vi "calculate Y ref.vi"(10 "Step size Y":dbl, 11 "Scan Index":i32) -> (2 "Next_Y_ref":dbl, 3 "Y_ref":dbl)   [LabVIEW 2014]
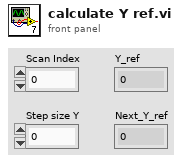
[diagram p1: front panel]
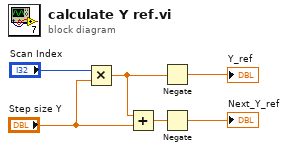
[diagram p0: block diagram]
diagram:
  n1 = Multiply(x="Scan Index", y="Step size Y") -> (x*y=w4:dbl)
  n2 = Add(x=w4, y="Step size Y") -> (x+y=w2:dbl)
  n3 = Negate(x=w4) -> (-x=→"Y_ref":dbl)
  n4 = Negate(x=w2) -> (-x=→"Next_Y_ref":dbl)
